vi "string_to_url.vi"(11 "string":string) -> (3 "url":string)   [LabVIEW 2015, in "lv-dropbox.lvlib"]
uses:
  lv-dropbox.lvlib
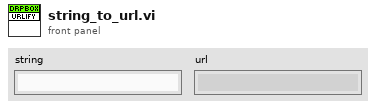
[diagram p1: front panel]
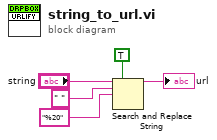
[diagram p0: block diagram]
diagram:
  n1 = Search and Replace String(replace all?=TRUE ("replace all? (F)"), input string="string", search string=" ", replace string="%20" ("replace string (\"\")")) -> (result string=→"url":string)  [unwired: 4 in, 3 out]
